vi "Secondary GPad.vi"() -> (14 "Turn?":bool, 16 "Fire?":bool, 17 "Repelling Balls?":bool, 18 "Right Side?":bool, 19 "Collecting Balls?":bool, 20 "Viewer Select":T2(ring)=enum."Ball Camera", 21 "Hoop Select":T1(ring), 22 "Number Of Balls":i32, 23 "Shooting Manual Override?":bool, 24 "Ball Managment Manual Override?":bool, 25 "No Target Alert":bool, 26 "Manual Override Engaged?":bool, 27 "Aligning?":bool)   [LabVIEW 2011]
uses:
  Team Code/Robot Global Data.vi
panel:
  in  "Distance Factor":dbl=0.5
  in  "Top Line":dbl=80.0
  in  "Bottom Line":dbl=140.0
  out "Hoop":enum32{"Top Hoop", "Bottom Hoop", "Mid Hoop"}(ring)
  out "Current RPM":dbl
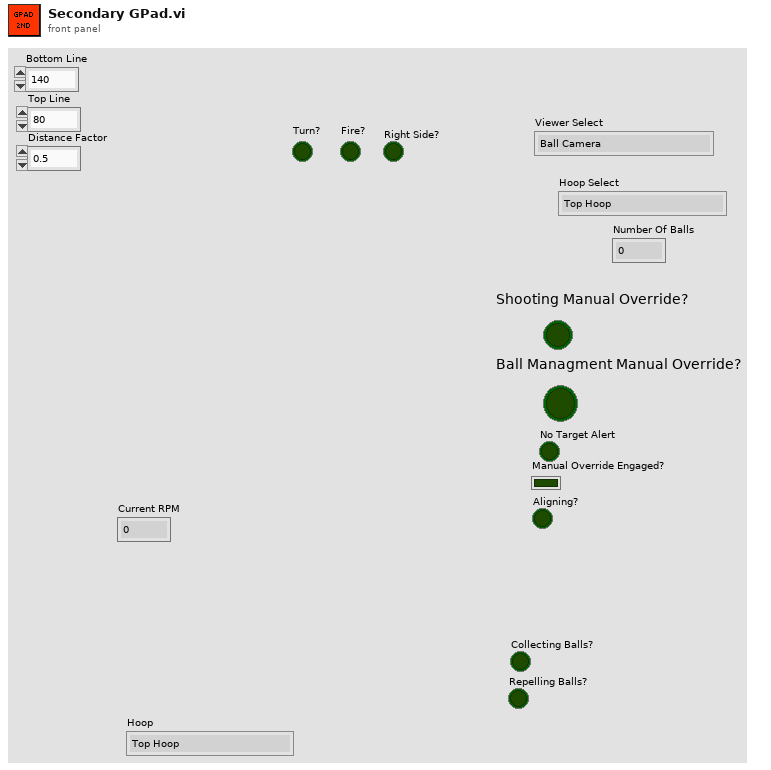
[diagram p1: front panel]
types:
  T1 = enum32{"Top Hoop", "Bottom Hoop", "Left Hoop", "Right Hoop"}
  T2 = enum32{"Target Camera", "Target Camera Mask", "Ball Camera", "Kinect Skeleton"}
  T3 = typedef "WPI_JoystickButtonState.ctl" = cluster{"Button 1":bool, "Button 2":bool, "Button 3":bool, "Button 4":bool, "Button 5":bool, "Button 6":bool, "Button 7":bool, "Button 8":bool, "Button 9":bool, "Button 10":bool, "Button 11":bool, "Button 12":bool}
  T4 = cluster{"Buttons":T3, "Axes":cluster{"axis 1 (x)":dbl, "axis 2 (y)":dbl, "axis 3 (throttle)":dbl, "axis 4":dbl, "axis 5":dbl, "axis 6":dbl}}
  T5 = cluster{"Position":cluster{"X Angle":dbl, "Raw Y":dbl, "Raw X":dbl}, "Distance (ft)":dbl, "BB Angle":dbl}
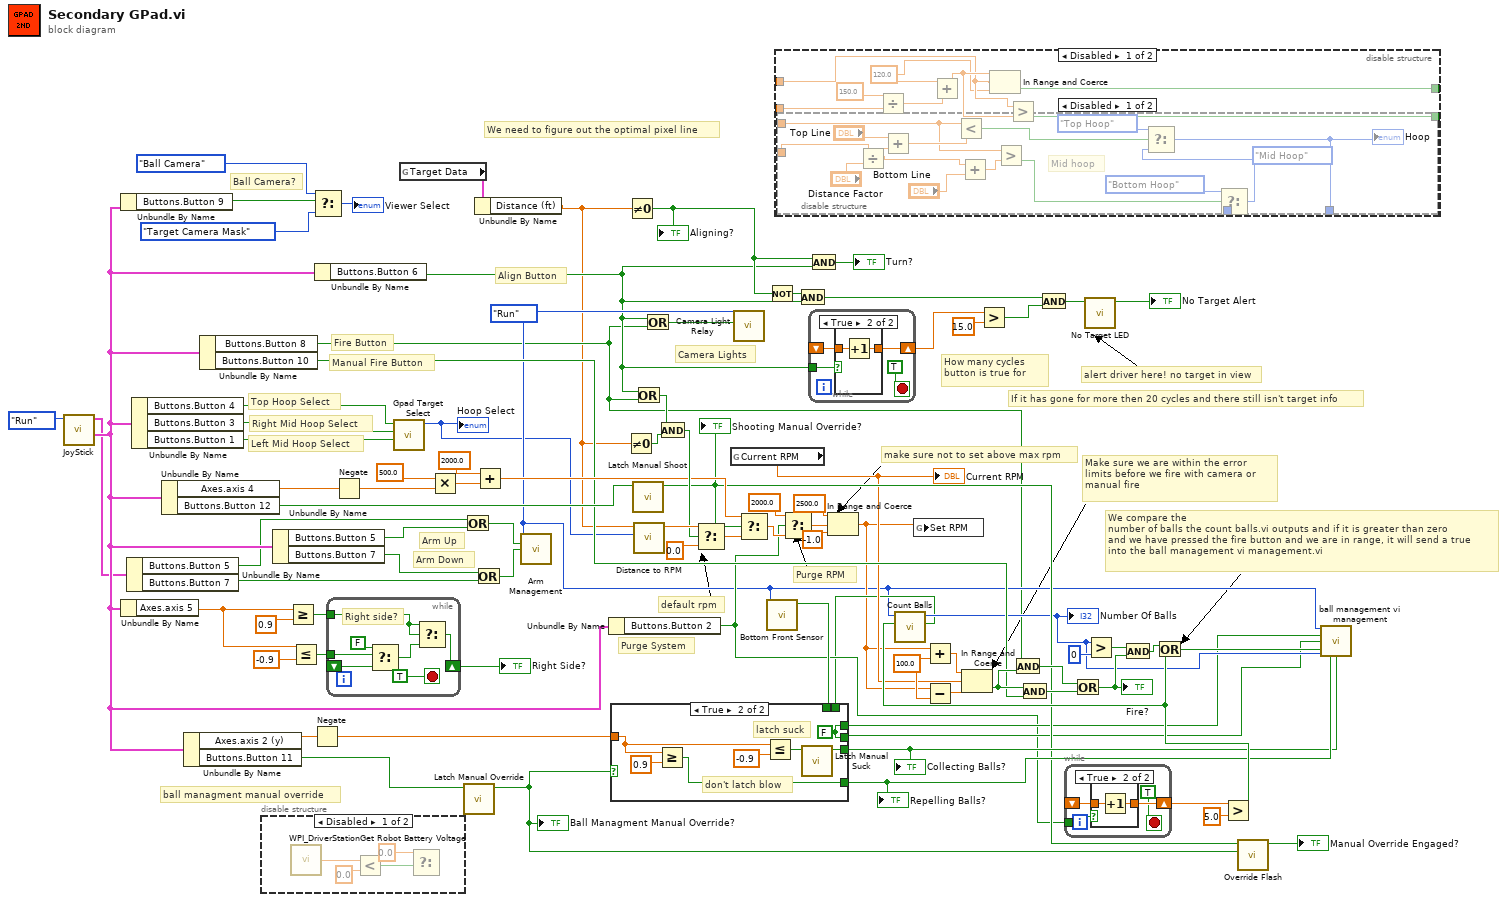
[diagram p0: block diagram]
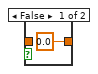
[diagram p5: hidden frame]
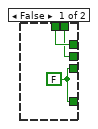
[diagram p6: hidden frame]
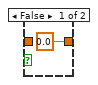
[diagram p7: hidden frame]
diagram:
  w74 = 100.0 ("y")
  w14 = enum16{"Init", "Run", "End"}."Run" ("Enum")
  # "default rpm"
  # "Make sure we are within the error limits before we fire with camera or manual fire"
  # "make sure not to set above max rpm"
  # "Purge System"
  # "Left Mid Hoop Select"
  # "Right Mid Hoop Select"
  # "Top Hoop Select"
  # "Purge RPM"
  # "We compare the \nnumber of balls the count balls.vi outputs and if it is greater than zero \nand we have pressed the fire button and we are in range, it will send a true\ninto the ball management vi management.vi"
  # "ball managment manual override"
  # "We need to figure out the optimal pixel line"
  # "Arm Down"
  # "Arm Up"
  # "Ball Camera?"
  # "Fire Button"
  # "Manual Fire Button"
  # "Camera Lights"
  # "Align Button"
  # "If it has gone for more then 20 cycles and there still isn't target info"
  # "How many cycles button is true for"
  # "alert driver here! no target in view"
  n1 = call "JoyStick.vi"("Enum"=enum16{"Init", "Run", "End"}."Run") -> ("JoyStick 3"=w34:T4, "JoyStick 1"=w13:T4)  [unwired: 7 in, 2 out]
  n2 = Unbundle By Name(w34) -> ("Buttons.Button 9"=w63:bool)
  n3 = Unbundle By Name(w34) -> ("Axes.axis 5"=w61:dbl)
  n4 = Unbundle By Name(w13) -> ("Buttons.Button 5"=w4:bool, "Buttons.Button 7"=w10:bool)
  n5 = Unbundle By Name(w34) -> ("Buttons.Button 4"=w40:bool, "Buttons.Button 3"=w69:bool, "Buttons.Button 1"=w68:bool)
  n6 = Unbundle By Name(w34) -> ("Axes.axis 4"=w56:dbl, "Buttons.Button 12"=w35:bool)
  n7 = Unbundle By Name(w34) -> ("Axes.axis 2 (y)"=w32:dbl, "Buttons.Button 11"=w33:bool)
  n8 = Unbundle By Name(w34) -> ("Buttons.Button 8"=w2:bool, "Buttons.Button 10"=w27:bool)
  n9 = disable-structure shown="Disabled" {
    frame Disabled {
      n10 = call <vilib>:"WPI_DriverStationGet Robot Battery Voltage.vi"() -> ("robot battery voltage"=w91:dbl)  [unwired: 14 in, 1 out]
      n11 = Less?(x=w91, y=0.0) -> (x < y?=w89:bool)
      n12 = Select(t=0.0, s=w89) -> ()  [unwired: 1 in, 1 out]
    }
    frame Enabled {
    }
  }
  n13 = Unbundle By Name(w34) -> ("Buttons.Button 5"=w5:bool, "Buttons.Button 7"=w9:bool)
  n14 = Greater Or Equal?(x=w61, y=0.9) -> (x >= y?=w59:bool)
  n15 = Less Or Equal?(x=w61, y=-0.9) -> (x <= y?=w58:bool)
  n16 = Negate(x=w32) -> (-x=w41:dbl)
  n17 = Select(t=T2."Ball Camera" ("Viewer Select"), s=w63, f=T2."Target Camera Mask" ("Viewer Select")) -> (s? t:f=→"Viewer Select":T2)
  n18 = Unbundle By Name(w34) -> ("Buttons.Button 6"=w8:bool)
  n19 = while {
    tunnel: w59 -> [w94]
    tunnel: w58 -> [w95]
    shift-right: [w96] -> w57
    shift-left: _ -> [w97]
    stop <- TRUE stop-if-true
    # "Right side?"
    n20 = Select(t=FALSE, s=w95, f=w97) -> (s? t:f=w98:bool)
    n21 = Select(t=w94, s=w94, f=w98) -> (s? t:f=w96:bool)
  }
  "Right Side?" <- w57
  n22 = Negate(x=w56) -> (-x=w42:dbl)
  n23 = call "Gpad Target Select.vi"("Left Hoop"=w68, "Right Hoop"=w69, "Top Hoop"=w40) -> ("Hoop Select"=w6:T1)  [unwired: 8 in]
  "Hoop Select" <- w6
  n24 = global read "Robot Global Data.vi" "Target Data"() -> (w30:T5)
  n25 = Multiply(x=500.0, y=w42) -> (x*y=w54:dbl)
  n26 = Or(x=w4, y=w5) -> (x .or. y?=w12:bool)
  n27 = call "Latch Manual Override.vi"("Input"=w33) -> ("Latched"=w48:bool)  [unwired: 10 in]
  "Ball Managment Manual Override?" <- w48
  n28 = Or(x=w9, y=w10) -> (x .or. y?=w11:bool)
  n29 = Unbundle By Name(w30) -> ("Distance (ft)"=w1:dbl)
  n30 = Add(x=2000.0, y=w54) -> (x+y=w52:dbl)
  n31 = call "Arm Management.vi"("Enum"=w14, "Up Button"=w12, "Down Button"=w11) -> ()  [unwired: 13 in]
  n32 = Unbundle By Name(w34) -> ("Buttons.Button 2"=w17:bool)
  n33 = Not Equal To 0?(x=w1) -> (x != 0?=w80:bool)
  n34 = Not Equal To 0?(x=w1) -> (x != 0?=w37:bool)
  "Aligning?" <- w37
  n35 = call "Latch Manual Shoot.vi"("Input"=w35) -> ("Latched"=w25:bool)  [unwired: 10 in]
  "Shooting Manual Override?" <- w25
  n36 = Or(x=w8, y=w2) -> (x .or. y?=w7:bool)
  n37 = call "Distance to RPM.vi"("Distance"=w1, "Hoop"=w6) -> ("Shooter RPM"=w84:dbl)  [unwired: 8 in]
  n38 = Or(x=w8, y=w2) -> (x .or. y?=w64:bool)
  n39 = And(x=w7, y=w80) -> (x .and. y?=w79:bool)
  n40 = Select(t=w84, s=w79, f=0.0) -> (s? t:f=w77:dbl)
  n41 = global read "Robot Global Data.vi" "Current RPM"() -> (w18:dbl)
  "Current RPM" <- w18
  n42 = call "Camera Light Relay.vi"("Camera Light"=w64, "Enum"=w14) -> ()  [unwired: 10 in]
  n43 = Select(t=w52, s=w25, f=w77) -> (s? t:f=w45:dbl)
  n44 = Not(x=w37) -> (.not. x?=w86:bool)
  n45 = call "Bottom Front Sensor.vi"("Enum"=w14) -> ("Bottom Front"=w24:bool)  [unwired: 10 in]
  n46 = disable-structure shown="Disabled" {
    disable-tunnel: _ -> [w104 _]
    disable-tunnel: [w103 _] -> _
    disable-tunnel: [w102 _] -> _
    disable-tunnel: _ -> [w100 _]
    frame Disabled {
      w99 = 120.0 ("y")
      n47 = disable-structure shown="Disabled" {
        disable-tunnel: _ -> [w120 _]
        disable-tunnel: [w117 _] -> _
        disable-tunnel: _ -> [w111 _]
        disable-tunnel: _ -> [w107 _]
        frame Disabled {
          (unwired) enum32{"Top Hoop", "Bottom Hoop", "Mid Hoop"}."Mid Hoop" ("Hoop")
          # "Mid hoop"
          n48 = Divide(x=w107, y="Distance Factor") -> (x/y=w110:dbl)
          n49 = Add(x="Top Line", y=w110) -> (x+y=w114:dbl)
          n50 = Less?(x=w111, y=w114) -> (x < y?=w115:bool)
          n51 = Add(x=w110, y="Bottom Line") -> (x+y=w108:dbl)
          n52 = Greater?(x=w111, y=w108) -> (0:w116:bool)
          n53 = Select(t=enum32{"Top Hoop", "Bottom Hoop", "Mid Hoop"}."Bottom Hoop" ("Hoop"), s=w116, f=w120) -> (s? t:f=w118:enum32{"Top Hoop", "Bottom Hoop", "Mid Hoop"})
          n54 = Select(t=enum32{"Top Hoop", "Bottom Hoop", "Mid Hoop"}."Top Hoop" ("Hoop"), s=w115, f=w118) -> (s? t:f=w117:enum32{"Top Hoop", "Bottom Hoop", "Mid Hoop"})
          "Hoop" <- w117
        }
        frame Enabled {
        }
      }
      n55 = Divide(x=150.0 ("y"), y=w104) -> (x/y=w105:dbl)
      n56 = Add(x=w99, y=w105) -> (x+y=w101:dbl)
      n57 = In Range and Coerce(upper limit=w101, x=w100, lower limit=w99) -> (In Range?=w103:bool)  [unwired: 1 out]
      n58 = Greater?(x=w100, y=w101) -> (0:w102:bool)
    }
    frame Enabled {
    }
  }
  n59 = Select(t=2000.0, s=w17, f=w45) -> (s? t:f=w44:dbl)
  n60 = And(x=w86, y=w8) -> (x .and. y?=w81:bool)
  n61 = And(x=w37, y=w8) -> (x .and. y?=→"Turn?":bool)
  n62 = while {
    tunnel: w8 -> [w125]
    shift-right: [w123] -> w82
    shift-left: _ -> [w124]
    stop <- TRUE stop-if-true
    n63 = case shown="True" w125 {
      tunnel: w124 -> [_ w128]
      tunnel: [0.0 w127] -> w123
      frame False {
      }
      frame True {
        n64 = Increment(x=w128) -> (x+1=w127:dbl)
      }
    }
  }
  n65 = In Range and Coerce(upper limit=2500.0, x=w44, lower limit=-1.0) -> (coerced(x)=w15:dbl)  [unwired: 1 out]
  n66 = global write "Robot Global Data.vi" "Set RPM"(w15) -> ()
  n67 = Add(x=w15, y=w74) -> (x+y=w73:dbl)
  n68 = Subtract(x=w15, y=w74) -> (x-y=w72:dbl)
  n69 = In Range and Coerce(upper limit=w73, x=w18, lower limit=w72) -> (In Range?=w71:bool)  [unwired: 1 out]
  n70 = Greater?(x=w82, y=15.0) -> (0:w36:bool)
  n71 = And(x=w2, y=w71) -> (x .and. y?=w76:bool)
  n72 = And(x=w71, y=w27) -> (x .and. y?=w75:bool)
  n73 = And(x=w81, y=w36) -> (x .and. y?=w3:bool)
  n74 = while {
    tunnel: w17 -> [w132]
    shift-right: [w130] -> w43
    shift-left: _ -> [w131]
    stop <- TRUE stop-if-true
    n75 = case shown="True" w132 {
      tunnel: w131 -> [_ w135]
      tunnel: [0.0 w134] -> w130
      frame False {
      }
      frame True {
        n76 = Increment(x=w135) -> (x+1=w134:dbl)
      }
    }
  }
  n77 = Or(x=w76, y=w75) -> (x .or. y?=w67:bool)
  "Fire?" <- w67
  n78 = call "No Target LED.vi"("Thing 1"=w3) -> ("Flashy the LED"=→"No Target Alert":bool)  [unwired: 10 in]
  n79 = Greater?(x=w43, y=5.0) -> (0:w29:bool)
  n80 = call "Count Balls.vi"("Reset Ball Count?"=w29, "Mode"=w14) -> ("Bottom Back?"=w16:bool, "Number Of Balls"=w23:i32)  [unwired: 8 in]
  "Number Of Balls" <- w23
  n81 = case shown="True" w48 {
    tunnel: w41 -> [_ w143]
    tunnel: w24 -> [w137 _]
    tunnel: [w138 w142] -> w28
    tunnel: [w138 w141] -> w26
    tunnel: [w137 w139] -> w22
    tunnel: w16 -> [w136 _]
    tunnel: [w136 w139] -> w21
    frame False {
      w138 = FALSE
    }
    frame True {
      w139 = FALSE ("Run Conveyor Feeder?")
      # "latch suck"
      # "don't latch blow"
      n82 = Greater Or Equal?(x=w143, y=0.9) -> (x >= y?=w142:bool)
      n83 = Less Or Equal?(x=w143, y=-0.9 ("x")) -> (x <= y?=w140:bool)
      n84 = call "Latch Manual Suck.vi"("Input"=w140) -> ("Latched"=w141:bool)  [unwired: 10 in]
    }
  }
  "Collecting Balls?" <- w26
  "Repelling Balls?" <- w28
  n85 = Greater?(x=w23, y=0) -> (0:w65:bool)
  n86 = And(x=w65, y=w67) -> (x .and. y?=w50:bool)
  n87 = Or(x=w50, y=w29) -> (x .or. y?=w51:bool)
  n88 = call "Override Flash.vi"("Thing 2"=w48, "Thing 1"=w25) -> ("Flashy the LED"=→"Manual Override Engaged?":bool)  [unwired: 9 in]
  n89 = call "ball management vi management.vi"("Enum"=w14, "Bottom Front Sensor"=w22, "Bottom Back Sensor"=w21, "Shoot?"=w51, "# of Balls"=w23, "Manual Blow Hard?"=w28, "Manual SUCK-IT HARD!!!!"=w26) -> ()  [unwired: 9 in]
